vi "Update CPU Graph.vi"(8 "error in (no error)":errorcluster, 9 "df":dbl, 10 "Plot":sgl[](array[numeric]), 11 "Simple UI in":refnum<class "Simple UI.lvclass">) -> (0 "error out":errorcluster, 3 "Simple UI out":refnum<class "Simple UI.lvclass">)   [LabVIEW 2020, in "Simple UI.lvlib" / "Simple UI.lvclass"]
uses:
  Simple UI.lvclass
  Simple UI.lvclass/Simple UI.ctl
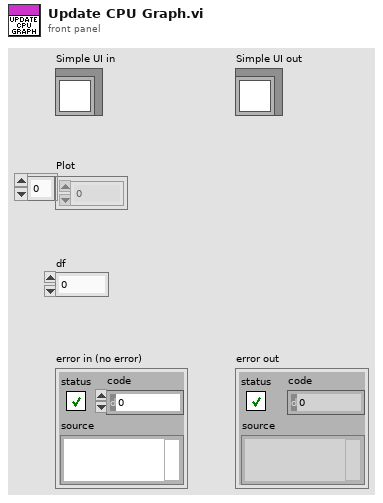
[diagram p1: front panel]
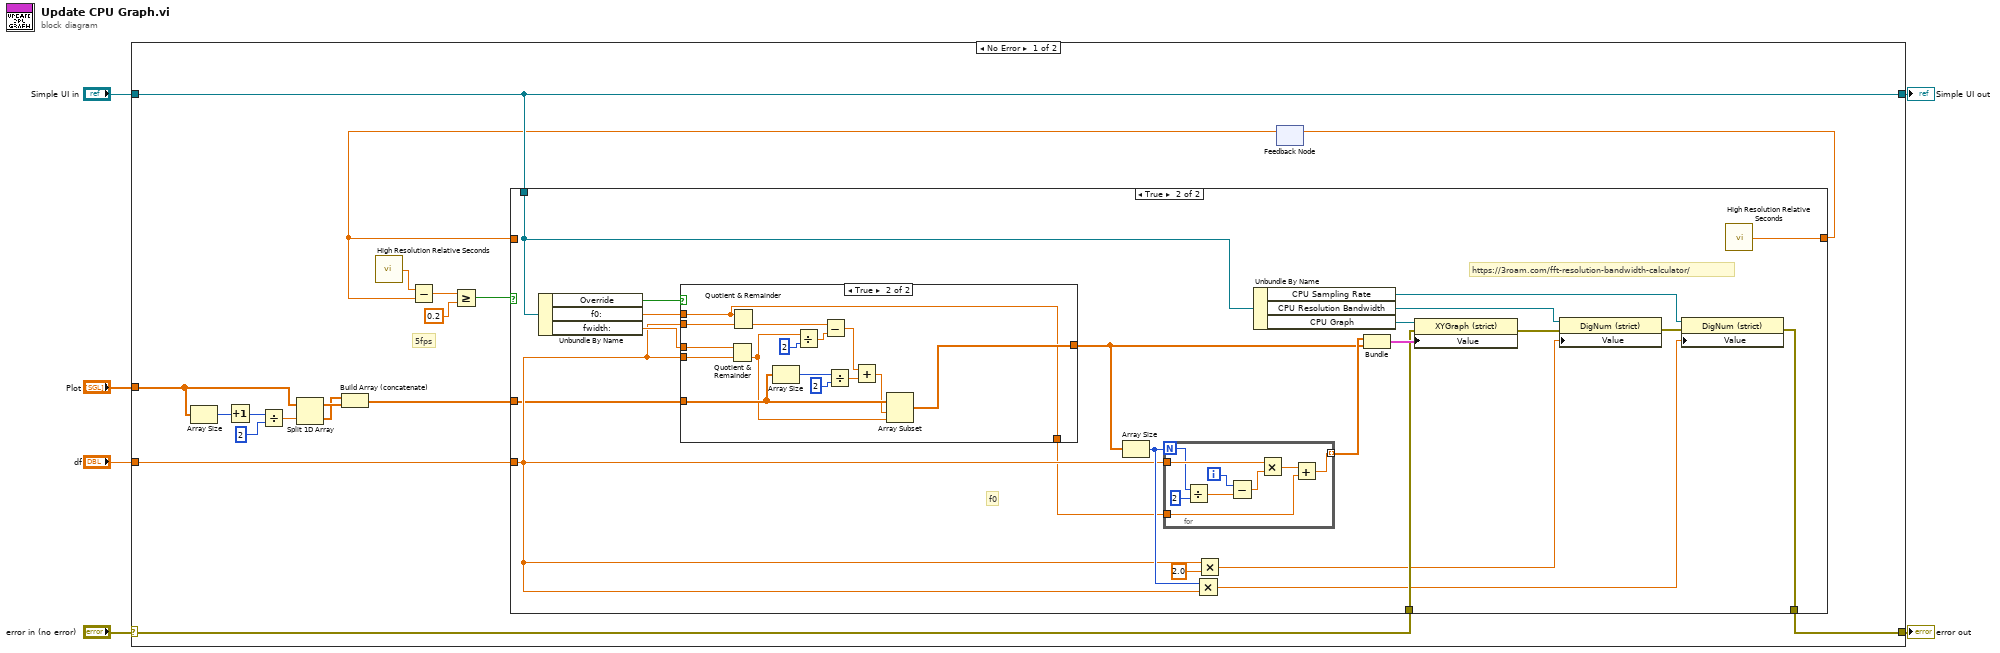
[diagram p0: block diagram]
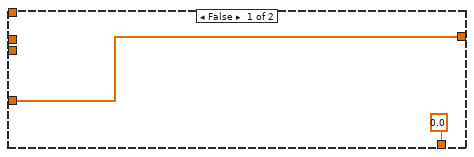
[diagram p3: hidden frame]
diagram:
  n1 = case shown="No Error" "error in (no error)" {
    selector: "error in (no error)" -> [w24 w76]
    tunnel: [w23 w76] -> w5
    tunnel: [w22 w75] -> w3
    tunnel: "Simple UI in" -> [w22 w75]
    tunnel: "Plot" -> [w8 _]
    tunnel: "df" -> [w21 _]
    frame No Error {
      # "5fps"
      n2 = Array Size(array=w8) -> (size(s)=w14:i32)
      n3 = Increment(x=w14) -> (x+1=w12:i32)
      n4 = Divide(x=w12, y=2) -> (x/y=w13:dbl)
      n5 = Split 1D Array(array=w8, index=w13) -> (first subarray=w10:sgl[], second subarray=w9:sgl[])
      n6 = Build Array (concatenate)(w9, w10) -> (w7:sgl[])
      n7 = call <vilib>:"High Resolution Relative Seconds.vi"() -> ("relative seconds"=w19:dbl)
      n8 = feedback #1() -> (w18:dbl)  [unwired: 1 in]
      n9 = Subtract(x=w19, y=w18) -> (x-y=w17:dbl)
      n10 = Greater Or Equal?(x=w17, y=0.2) -> (x >= y?=w16:bool)
      n11 = case shown="True" w16 {
        tunnel: w24 -> [w25 w46]
        tunnel: [w25 w40] -> w23
        tunnel: w22 -> [_ w37]
        tunnel: w21 -> [_ w33]
        tunnel: w7 -> [_ w31]
        tunnel: [w26 w29] -> w20
        tunnel: w18 -> [w26 _]
        frame False {
        }
        frame True {
          # "f0"
          # "https://3roam.com/fft-resolution-bandwidth-calculator/"
          n12 = Unbundle By Name(w37) -> ("Override"=w35:bool, "f0:"=w36:dbl, "fwidth:"=w34:dbl)
          n13 = case shown="True" w35 {
            tunnel: w36 -> [_ w51]
            tunnel: w34 -> [_ w65]
            tunnel: w33 -> [_ w64]
            tunnel: w33 -> [_ w63]
            tunnel: [w50 w62] -> w32
            tunnel: w31 -> [w50 w61]
            tunnel: [0.0 w51] -> w30
            frame False {
            }
            frame True {
              n14 = Quotient & Remainder(x=w65, y=w64) -> (floor(x/y)=w54:dbl)  [unwired: 1 out]
              n15 = Quotient & Remainder(x=w51, y=w63) -> (floor(x/y)=w59:dbl)  [unwired: 1 out]
              n16 = Array Size(array=w61) -> (size(s)=w60:i32)
              n17 = Divide(x=w54, y=2) -> (x/y=w52:dbl)
              n18 = Subtract(x=w59, y=w52) -> (x-y=w53:dbl)
              n19 = Divide(x=w60, y=2) -> (x/y=w56:dbl)
              n20 = Add(x=w53, y=w56) -> (x+y=w57:dbl)
              n21 = Array Subset(array=w61, index=w57, length=w54) -> (w62:sgl[])
            }
          }
          n22 = Array Size(array=w32) -> (size(s)=w38:i32)
          n23 = for {
            N: w38 -> [w73]
            tunnel: w33 -> [w74]
            tunnel: [w66] -> w48 mode=indexing
            tunnel: w30 -> [w69]
            i -> [w71]
            n24 = Divide(x=w73, y=2) -> (x/y=w70:dbl)
            n25 = Subtract(x=w71, y=w70) -> (x-y=w68:dbl)
            n26 = Multiply(x=w74, y=w68) -> (x*y=w67:dbl)
            n27 = Add(x=w67, y=w69) -> (x+y=w66:dbl)
          }
          n28 = Multiply(x=w38, y=w33) -> (x*y=w39:dbl)
          n29 = Multiply(x=w33, y=2.0) -> (x*y=w28:dbl)
          n30 = Unbundle By Name(w37) -> ("CPU Sampling Rate"=w41:refnum<vi>, "CPU Resolution Bandwidth"=w43:refnum<vi>, "CPU Graph"=w45:refnum<vi>)
          n31 = Bundle(w48, w32) -> (w47:cluster{dbl[], sgl[]})  [unwired: 1 in]
          n32 = property class="XYGraph (strict)"(reference=w45, error in=w46, "Value"=w47) -> (error out=w44:errorcluster)  [unwired: 1 out]
          n33 = property class="DigNum (strict)"(reference=w43, error in=w44, "Value"=w28) -> (error out=w42:errorcluster)  [unwired: 1 out]
          n34 = property class="DigNum (strict)"(reference=w41, error in=w42, "Value"=w39) -> (error out=w40:errorcluster)  [unwired: 1 out]
          n35 = call <vilib>:"High Resolution Relative Seconds.vi"() -> ("relative seconds"=w29:dbl)
        }
      }
      n36 = feedback-in #1(w20) -> ()
    }
    frame Error {
    }
  }
  "error out" <- w5
  "Simple UI out" <- w3
